vi "FRCts20_Backend_GetTeamStats.vi"(8 "error in (no error)":errorcluster) -> (0 "error out":errorcluster, 2 "Stats":T1)   [LabVIEW 2014, in "FRCts20_Backend_WebMethods.lvlib"]
doc: "The GetTeamStats function will return all calculated competition statistics from the data processor. Items include <b>software usage statistics</b>, <b>issue time averages</b>, and <b>daily resolution statistics</b>."
uses:
  FRCts20_Backend_WebMethods.lvlib
  FRCts20_Backend_FGVOperation.ctl
  FRCts20_Backend_Engine.lvlib
  FRCts20_Backend_NumTeams.ctl
  FRCts20_Backend_Controls.lvlib
  FRCts20_Backend_PercTeams.ctl
  FRCts20_Backend_SoftwareUsage.ctl
  FRCts20_Backend_ResPerDayPerQuad.ctl
  FRCts20_Backend_ResDayTotals.ctl
  FRCts20_Backend_ResQuadTotals.ctl
  FRCts20_Backend_Resolved.ctl
  FRCts20_Backend_OpenQuadTotals.ctl
  FRCts20_Backend_Open.ctl
  FRCts20_Backend_Issues.ctl
  FRCts20_Backend_Stats.ctl
panel:
  in  "Stats_Ref":T1
  # "The GetTeamStats function will return all\ncalculated competition statistics from the \ndata processor. Items include software\nusage statistics, issue time averages, and \ndaily resolution statistics."
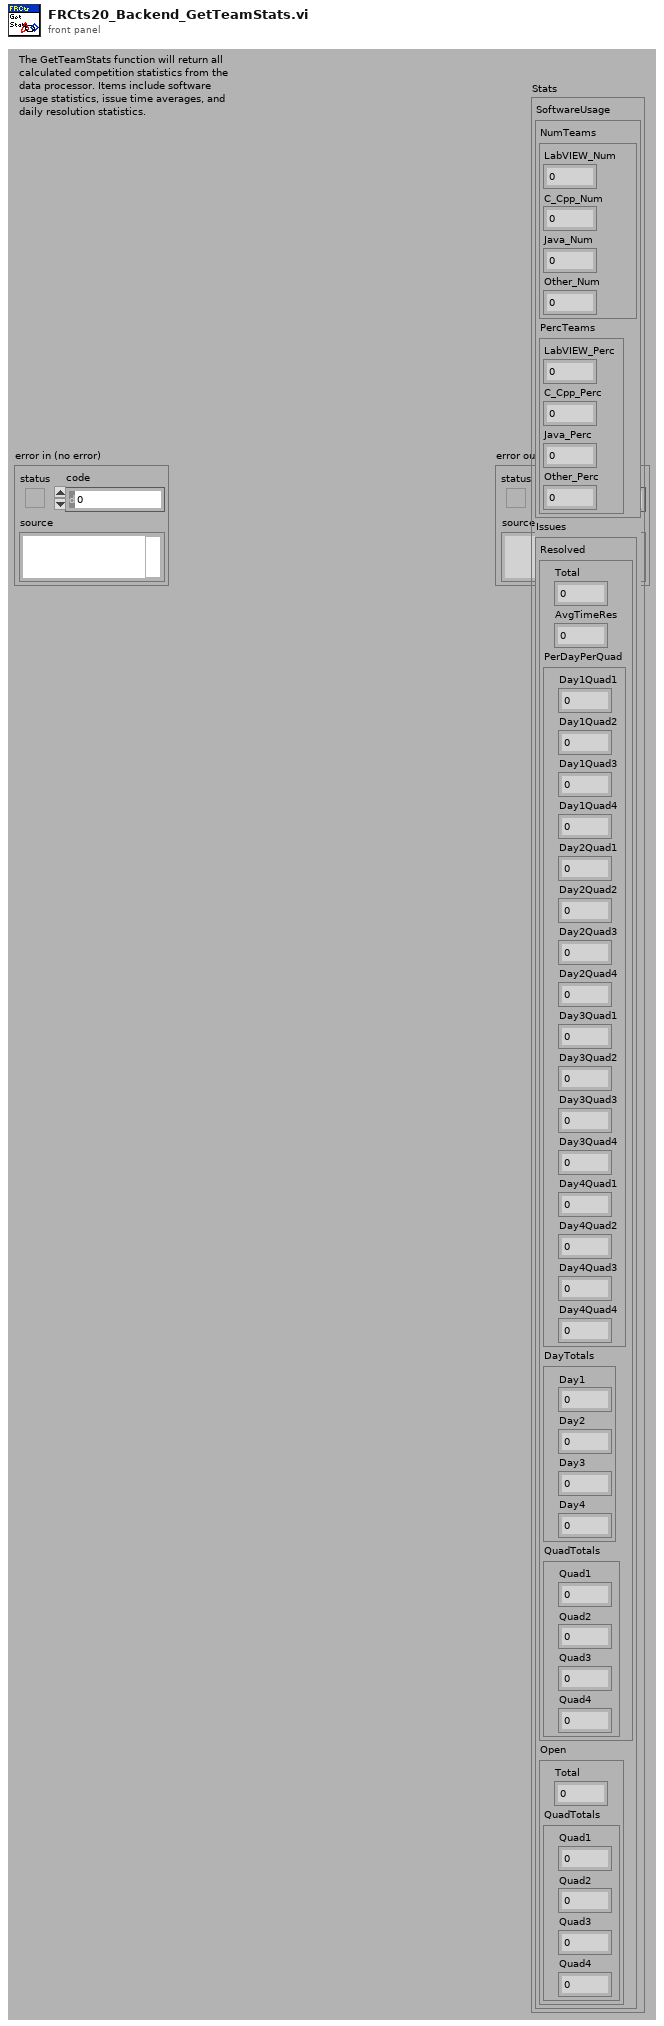
[diagram p1: front panel]
types:
  T1 = typedef "FRCts20_Backend_Controls.lvlib/FRCts20_Backend_Stats.ctl" = cluster{"SoftwareUsage":T2, "Issues":T5}
  T2 = typedef "FRCts20_Backend_Controls.lvlib/FRCts20_Backend_SoftwareUsage.ctl" = cluster{"NumTeams":T3, "PercTeams":T4}
  T3 = typedef "FRCts20_Backend_Controls.lvlib/FRCts20_Backend_NumTeams.ctl" = cluster{"LabVIEW_Num":u16, "C_Cpp_Num":u16, "Java_Num":u16, "Other_Num":u16}
  T4 = typedef "FRCts20_Backend_Controls.lvlib/FRCts20_Backend_PercTeams.ctl" = cluster{"LabVIEW_Perc":dbl, "C_Cpp_Perc":dbl, "Java_Perc":dbl, "Other_Perc":dbl}
  T5 = typedef "FRCts20_Backend_Controls.lvlib/FRCts20_Backend_Issues.ctl" = cluster{"Resolved":T6, "Open":T10}
  T6 = typedef "FRCts20_Backend_Controls.lvlib/FRCts20_Backend_Resolved.ctl" = cluster{"Total":u16, "AvgTimeRes":dbl, "PerDayPerQuad":T7, "DayTotals":T8, "QuadTotals":T9}
  T7 = typedef "FRCts20_Backend_Controls.lvlib/FRCts20_Backend_ResPerDayPerQuad.ctl" = cluster{"Day1Quad1":u16, "Day1Quad2":u16, "Day1Quad3":u16, "Day1Quad4":u16, "Day2Quad1":u16, "Day2Quad2":u16, "Day2Quad3":u16, "Day2Quad4":u16, "Day3Quad1":u16, "Day3Quad2":u16, "Day3Quad3":u16, "Day3Quad4":u16, "Day4Quad1":u16, "Day4Quad2":u16, "Day4Quad3":u16, "Day4Quad4":u16}
  T8 = typedef "FRCts20_Backend_Controls.lvlib/FRCts20_Backend_ResDayTotals.ctl" = cluster{"Day1":u16, "Day2":u16, "Day3":u16, "Day4":u16}
  T9 = typedef "FRCts20_Backend_Controls.lvlib/FRCts20_Backend_ResQuadTotals.ctl" = cluster{"Quad1":u16, "Quad2":u16, "Quad3":u16, "Quad4":u16}
  T10 = typedef "FRCts20_Backend_Controls.lvlib/FRCts20_Backend_Open.ctl" = cluster{"Total":u16, "QuadTotals":T11}
  T11 = typedef "FRCts20_Backend_Controls.lvlib/FRCts20_Backend_OpenQuadTotals.ctl" = cluster{"Quad1":u16, "Quad2":u16, "Quad3":u16, "Quad4":u16}
  T12 = typedef "FRCts20_Backend_Engine.lvlib/FRCts20_Backend_FGVOperation.ctl" = enum16{"Initialize", "EnqueueMessage", "EnqueueDataReturn", "FlushMessage", "FlushDataReturn"}
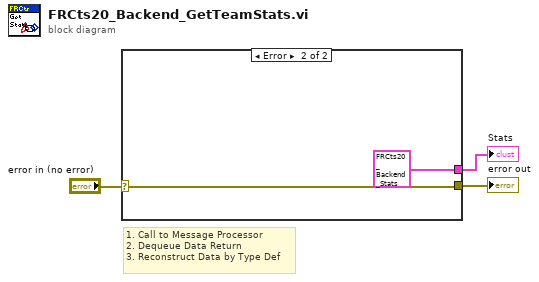
[diagram p0: block diagram]
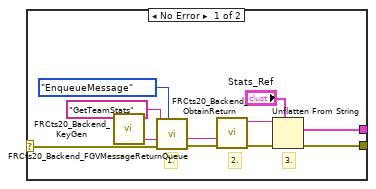
[diagram p2: hidden frame]
diagram:
  # "1. Call to Message Processor\n2. Dequeue Data Return\n3. Reconstruct Data by Type Def"
  n1 = case shown="Error" "error in (no error)" {
    selector: "error in (no error)" -> [w14 w16]
    tunnel: [w8 w16] -> w2
    tunnel: [w6 T1 {"SoftwareUsage"={"NumTeams"={"LabVIEW_Num"=0, "C_Cpp_Num"=0, "Java_Num"=0, "Other_Num"=0}, "PercTeams"={"LabVIEW_Perc"=0.0, "C_Cpp_Perc"=0.0, "Java_Perc"=0.0, "Other_Perc"=0.0}}, "Issues"={"Resolved"={"Total"=0, "AvgTimeRes"=0.0, "PerDayPerQuad"={"Day1Quad1"=0, "Day1Quad2"=0, "Day1Quad3"=0, "Day1Quad4"=0, "Day2Quad1"=0, "Day2Quad2"=0, "Day2Quad3"=0, "Day2Quad4"=0, "Day3Quad1"=0, "Day3Quad2"=0, "Day3Quad3"=0, "Day3Quad4"=0, "Day4Quad1"=0, "Day4Quad2"=0, "Day4Quad3"=0, "Day4Quad4"=0}, "DayTotals"={"Day1"=0, "Day2"=0, "Day3"=0, "Day4"=0}, "QuadTotals"={"Quad1"=0, "Quad2"=0, "Quad3"=0, "Quad4"=0}}, "Open"={"Total"=0, "QuadTotals"={"Quad1"=0, "Quad2"=0, "Quad3"=0, "Quad4"=0}}}} ("Stats_Ref")] -> w1
    frame No Error {
      # "3."
      # "2."
      # "1."
      n2 = call "FRCts20_Backend_KeyGen.vi"() -> ("Keygen"=w11:string)  [unwired: 27 in]
      n3 = call "FRCts20_Backend_FGVMessageReturnQueue.vi"("Operation"=FRCts20_Backend_FGVOperation."EnqueueMessage", "error in (no error)"=w14, "Key"=w11, "Message Name"="GetTeamStats") -> ("error out"=w10:errorcluster, "Key (Duplicate)"=w5:string)  [unwired: 4 in]
      n4 = call "FRCts20_Backend_ObtainReturn.vi"("error in (no error)"=w10, "Key"=w5) -> ("error out"=w9:errorcluster, "Message Value"=w4:string)  [unwired: 8 in]
      n5 = Unflatten From String(type="Stats_Ref", binary string=w4, error in (no error)=w9) -> (value=w6:T1, error out=w8:errorcluster)  [unwired: 2 in, 1 out]
    }
    frame Error {
    }
  }
  "error out" <- w2
  "Stats" <- w1
